vi "Configure Slew Rate Trigger Src.vi"(0 "VISA Resource Name":refnum<visa-resource-name>, 1 "Delta Time (1.0e-9 s)":dbl=1e-09 format="%.2p", 2 "High Threshold (0.0 V)":dbl format="%.2p", 5 "Trigger Source (Channel 1)":string(combo)="CH1", 7 "Polarity (Either)":i32(slide)=3, 9 "Trigger When (Faster than)":i32(slide)=1, 11 "error in (no error)":errorcluster {"code" format="%.0x"}, 12 "Low Threshold (0.0 V)":dbl format="%.2p") -> (4 "VISA Resource Name Out":refnum<visa-resource-name>, 15 "error out":errorcluster {"code" format="%.0x"})   [LabVIEW 2010, in "Tektronix TDS 3000 Series.lvlib"]
doc: "This VI configures the scope for slew rate triggering. Slew rate triggering is often used to check the large signal response of amplifiers. When using slew rate triggering, the oscilloscope triggers on a pulse edge that has a slew rate faster or slower than the rate you specify. You specify whether the oscilloscope triggers on a positive or negative slew rate with the Polarity control. You specify whether the trigger looks for a slew rate faster or slower than the one you specify with the Trigger When control. You specify the delta type with the Delta Time control. You specify the high and low threshold values with the High Threshold and Low Threshold controls, respectively. The oscilloscope calculates the slew rate as follows.\n\n (High Threshold - Low Threshold) / Delta Time\n\n\nNotes:\n\n(1) This VI affects instrument behavior only if the Trigger Type is set to Slew Trigger. Call the Configure Trigger VI to set the Trigger Type before you call this VI."
uses:
  <instrlib>/Tektronix TDS 3000 Series/Tektronix TDS 3000 Series.lvlib
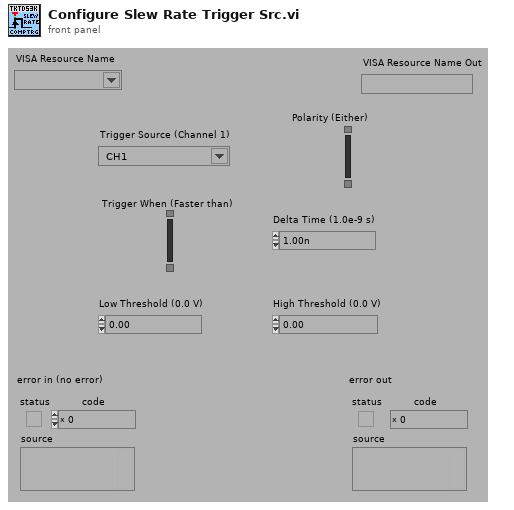
[diagram p1: front panel]
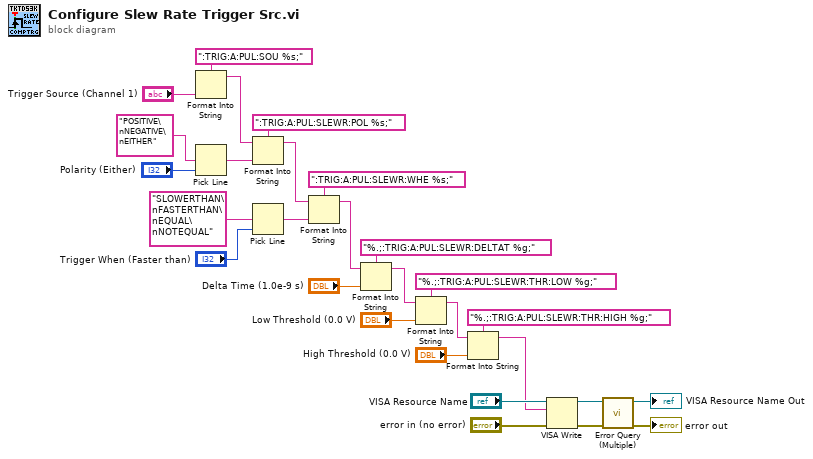
[diagram p0: block diagram]
diagram:
  n1 = Format Into String(format string=":TRIG:A:PUL:SOU %s;", "Trigger Source (Channel 1)") -> (resulting string=w20:string)  [unwired: 2 in, 1 out]
  n2 = Pick Line(multi-line string="POSITIVE\nNEGATIVE\nEITHER", line index="Polarity (Either)") -> (output string=w22:string)  [unwired: 1 in]
  n3 = Format Into String(format string=":TRIG:A:PUL:SLEWR:POL %s;", initial string=w20, w22) -> (resulting string=w10:string)  [unwired: 1 in, 1 out]
  n4 = Pick Line(multi-line string="SLOWERTHAN\nFASTERTHAN\nEQUAL\nNOTEQUAL", line index="Trigger When (Faster than)") -> (output string=w17:string)  [unwired: 1 in]
  n5 = Format Into String(format string=":TRIG:A:PUL:SLEWR:WHE %s;", initial string=w10, w17) -> (resulting string=w9:string)  [unwired: 1 in, 1 out]
  n6 = Format Into String(format string="%.;:TRIG:A:PUL:SLEWR:DELTAT %g;", initial string=w9, "Delta Time (1.0e-9 s)") -> (resulting string=w7:string)  [unwired: 1 in, 1 out]
  n7 = Format Into String(format string="%.;:TRIG:A:PUL:SLEWR:THR:LOW %g;", initial string=w7, "Low Threshold (0.0 V)") -> (resulting string=w6:string)  [unwired: 1 in, 1 out]
  n8 = Format Into String(format string="%.;:TRIG:A:PUL:SLEWR:THR:HIGH %g;", initial string=w6, "High Threshold (0.0 V)") -> (resulting string=w5:string)  [unwired: 1 in, 1 out]
  n9 = VISA Write(VISA resource name="VISA Resource Name", write buffer=w5, error in (no error)="error in (no error)") -> (VISA resource name out=w4:refnum<visa-resource-name>, error out=w3:errorcluster)  [unwired: 1 out]
  n10 = call <instrlib>:"Error Query (Multiple).vi"("error in (no error)"=w3, "VISA Resource Name"=w4) -> ("error out"=→"error out":errorcluster, "VISA Resource Name Out"=→"VISA Resource Name Out":refnum<visa-resource-name>)  [unwired: 6 in, 2 out]
